vi "Custom-Turn.vi"(8 "Wanted Angle":dbl, 11 "Wheel Angle":dbl) -> (3 "Mode":string)   [LabVIEW 2011]
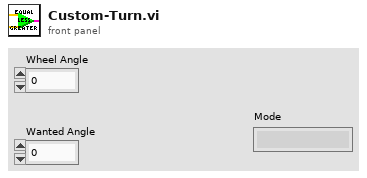
[diagram p1: front panel]
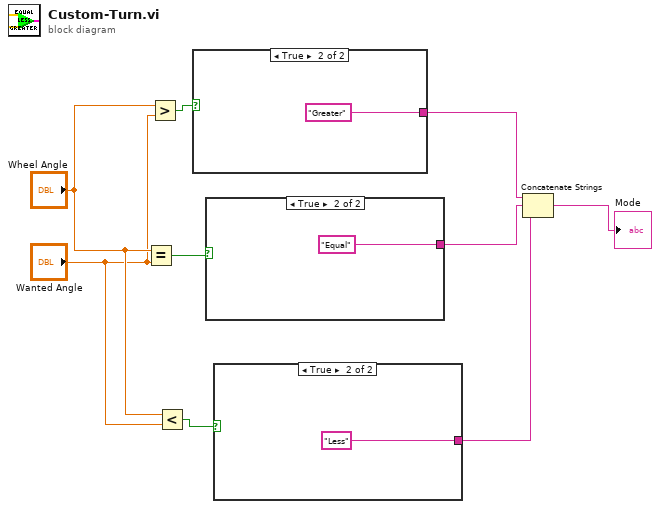
[diagram p0: block diagram]
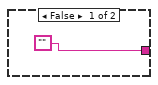
[diagram p2: hidden frame]
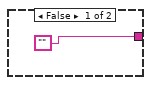
[diagram p3: hidden frame]
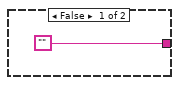
[diagram p4: hidden frame]
diagram:
  n1 = Equal?(x="Wheel Angle", y="Wanted Angle") -> (x = y?=w5:bool)
  n2 = Greater?(x="Wheel Angle", y="Wanted Angle") -> (0:w9:bool)
  n3 = Less?(x="Wheel Angle", y="Wanted Angle") -> (x < y?=w6:bool)
  n4 = case shown="True" w9 {
    tunnel: ["" "Greater"] -> w4
    frame False {
    }
    frame True {
    }
  }
  n5 = case shown="True" w5 {
    tunnel: ["" "Equal"] -> w3
    frame False {
    }
    frame True {
    }
  }
  n6 = case shown="True" w6 {
    tunnel: ["" "Less"] -> w2
    frame False {
    }
    frame True {
    }
  }
  n7 = Concatenate Strings(w4, w3, w2) -> (→"Mode":string)
